vi "Browser Core Tests.vi"(8 "error in (no error)":errorcluster) -> (0 "error out":errorcluster)   [LabVIEW 2017, in "Unit Tests.lvlib"]
uses:
  Unit Tests.lvlib
  <vilib>/addons/_JKI Toolkits/Caraya/classes/Test Suite/Test Suite.lvclass
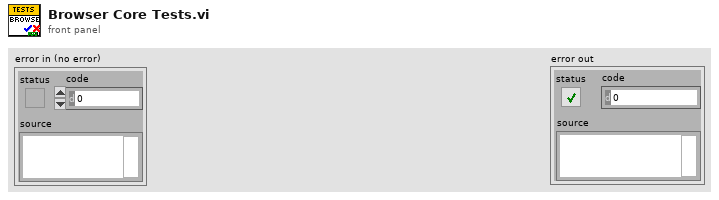
[diagram p1: front panel]
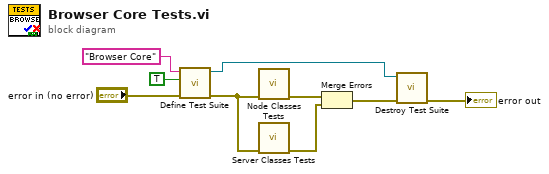
[diagram p0: block diagram]
diagram:
  n1 = call <vilib>:"Define Test Suite.vi"("error in (no error)"="error in (no error)", "Interactive"=TRUE, "Label (VI Title)"="Browser Core") -> ("error out"=w5:errorcluster, "Test Suite"=w2:refnum<class "Test Suite.lvclass">)  [unwired: 7 in]
  n2 = call "Node Classes Tests.vi"("error in (no error)"=w5) -> ("error out"=w9:errorcluster)  [unwired: 10 in]
  n3 = call "Server Classes Tests.vi"("error in (no error)"=w5) -> ("error out"=w8:errorcluster)  [unwired: 10 in]
  n4 = Merge Errors(w9, w8) -> (w3:errorcluster)
  n5 = call-dynamic "Destroy Test Suite.vi"("error in (no error)"=w3, "Test Suite in"=w2) -> ("error out"=→"error out":errorcluster)  [unwired: 9 in]
